vi "mathematics DAQ value.vi"(7 "Array":dbl[][](array[numeric])) -> (0 "Array 2":dbl[](array[numeric]), 1 "湿度?":dbl, 2 "温度?":dbl)   [LabVIEW 2012]
uses:
  <vilib>/Analysis/baseanly.llb/Mean (DBL).vi
  <vilib>/Analysis/NI_AALBase.lvlib
panel:
  out "数组 2":dbl[](array[numeric])
  out "数组":dbl[](array[numeric])
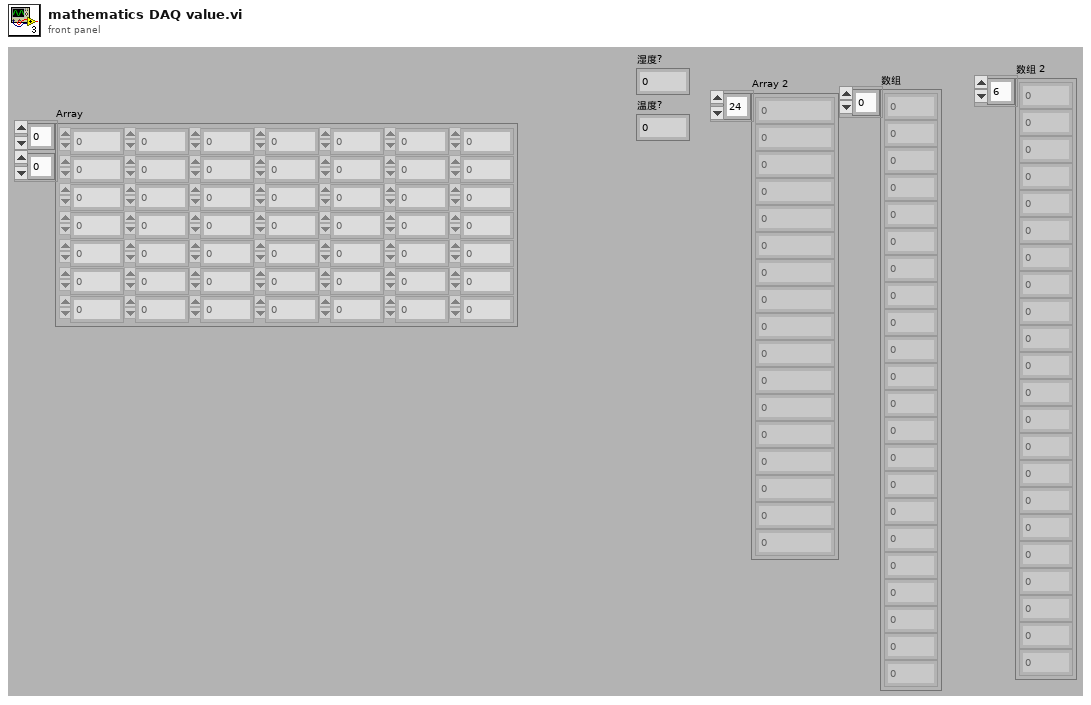
[diagram p1: front panel]
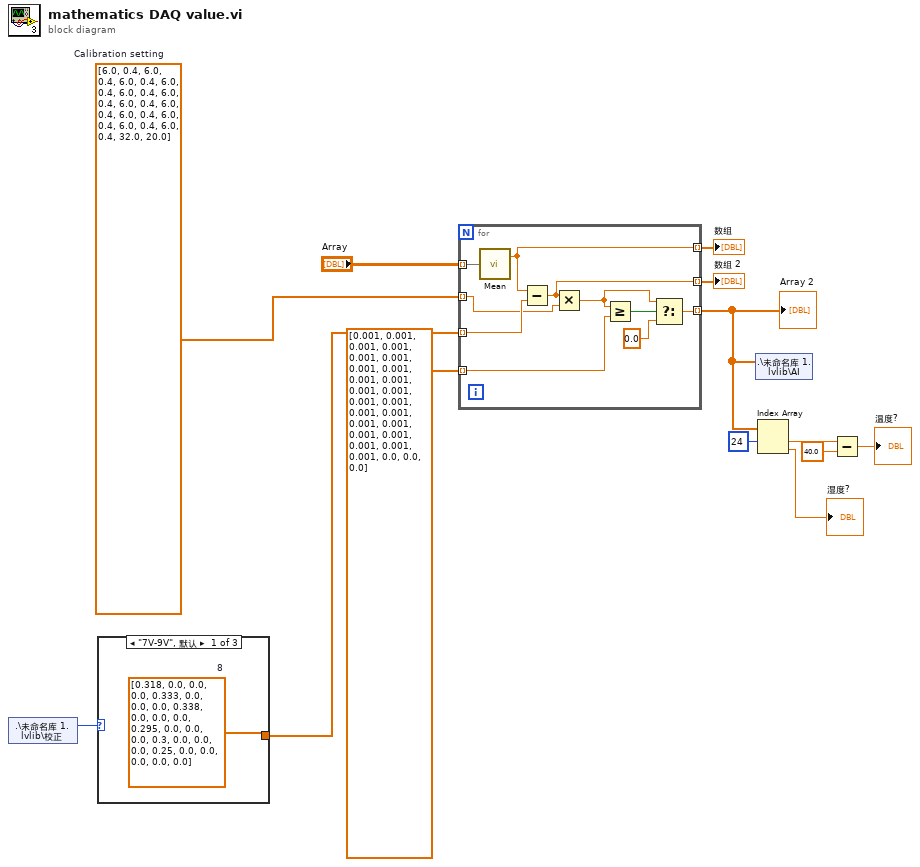
[diagram p0: block diagram]
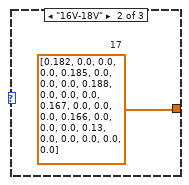
[diagram p2: hidden frame]
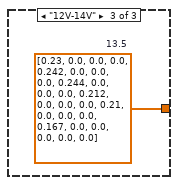
[diagram p3: hidden frame]
diagram:
  w12 = dbl[] [6.0, 0.4, 6.0, 0.4, 6.0, 0.4, 6.0, 0.4, 6.0, 0.4, 6.0, 0.4, 6.0, 0.4, 6.0, 0.4, 6.0, 0.4, 6.0, 0.4, 6.0, 0.4, 6.0, 0.4, 32.0, 20.0]  # Calibration setting
  n1 = shared-variable ".\\未命名库 1.lvlib\\校正"() -> (w8:enum16{"7V-9V", "12V-14V", "16V-18V"})  [unwired: 1 in, 1 out]
  n2 = case shown="\"7V-9V\", 默认" w8 {
    tunnel: [w14 w15 w16] -> w7
    frame "7V-9V", Default {
      w14 = dbl[] [0.318, 0.0, 0.0, 0.0, 0.333, 0.0, 0.0, 0.0, 0.338, 0.0, 0.0, 0.0, 0.295, 0.0, 0.0, 0.0, 0.3, 0.0, 0.0, 0.0, 0.25, 0.0, 0.0, 0.0, 0.0, 0.0]  # 8
    }
    frame "16V-18V" {
      w15 = dbl[] [0.182, 0.0, 0.0, 0.0, 0.185, 0.0, 0.0, 0.0, 0.188, 0.0, 0.0, 0.0, 0.167, 0.0, 0.0, 0.0, 0.166, 0.0, 0.0, 0.0, 0.13, 0.0, 0.0, 0.0, 0.0, 0.0]  # 17
    }
    frame "12V-14V" {
      w16 = dbl[] [0.23, 0.0, 0.0, 0.0, 0.242, 0.0, 0.0, 0.0, 0.244, 0.0, 0.0, 0.0, 0.212, 0.0, 0.0, 0.0, 0.21, 0.0, 0.0, 0.0, 0.167, 0.0, 0.0, 0.0, 0.0, 0.0]  # 13.5
    }
  }
  n3 = for {
    tunnel: "Array" -> [w21] mode=indexing
    tunnel: w12 -> [w20] mode=indexing
    tunnel: w7 -> [w22] mode=indexing
    tunnel: dbl[] [0.001, 0.001, 0.001, 0.001, 0.001, 0.001, 0.001, 0.001, 0.001, 0.001, 0.001, 0.001, 0.001, 0.001, 0.001, 0.001, 0.001, 0.001, 0.001, 0.001, 0.001, 0.001, 0.001, 0.0, 0.0, 0.0] ("Show lower setting") -> [w26] mode=indexing
    tunnel: [w23] -> w6 mode=indexing
    tunnel: [w18] -> w10 mode=indexing
    tunnel: [w17] -> w9 mode=indexing
    n4 = call-poly <vilib>:"Mean.vi"("X"=w21) -> ("mean"=w18:dbl)  [unwired: 1 out]
    n5 = Subtract(x=w18, y=w22) -> (x-y=w17:dbl)
    n6 = Multiply(x=w17, y=w20) -> (x*y=w19:dbl)
    n7 = Greater Or Equal?(x=w19, y=w26) -> (x >= y?=w25:bool)
    n8 = Select(t=w19, s=w25, f=0.0) -> (s? t:f=w23:dbl)
  }
  "Array 2" <- w6
  "数组" <- w10
  "数组 2" <- w9
  n9 = shared-variable ".\\未命名库 1.lvlib\\AI"(w6) -> ()  [unwired: 1 in, 1 out]
  n10 = Index Array(array=w6, index #1=24 ("索引")) -> (element #1=w4:dbl, element #2=→"湿度?":dbl)  [unwired: 1 in]
  n11 = Subtract(x=w4, y=40.0) -> (x-y=→"温度?":dbl)
